vi "Test-FAMM.vi"() -> ()   [LabVIEW 2014, in "FAMM.lvclass"]
doc: "Test the Historian performance"
uses:
  FAMM.lvclass
  HISW/HISW.lvclass
  FAMM.lvclass/FAMM.ctl
  Common/controls/GlobalClassRefs.vi
panel:
  out "Tags":i32
  out "error out":errorcluster
  out "Database Class":string
  out "FAMM_PAQ_Layers":i32
  out "37x37":picture
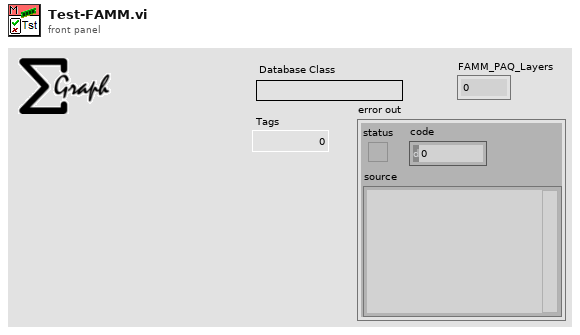
[diagram p1: front panel]
types:
  T1 = typedef "typedef_PAQsample.ctl" = cluster{"TAGs":string[], "status":u32[], "data":dbl[], "Source":string[]}
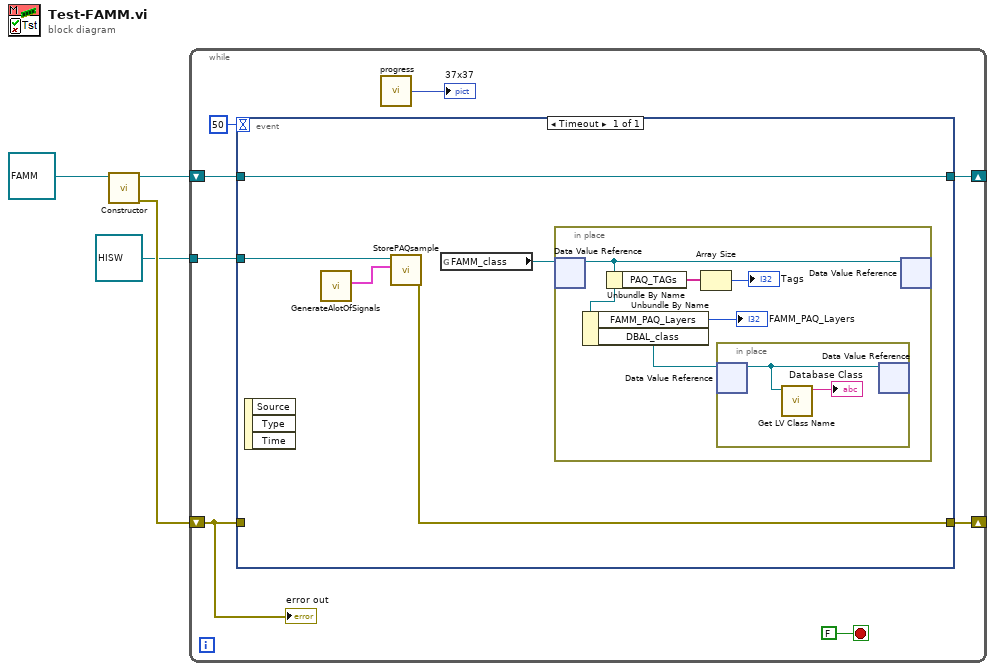
[diagram p0: block diagram]
diagram:
  n1 = call "Constructor.vi"("FAMM in"=refnum<class "FAMM.lvclass"> refnum) -> ("error out"=w4:errorcluster, "FAMM out"=w1:refnum<class "FAMM.lvclass">)  [unwired: 9 in]
  n2 = while {
    shift-right: [w9] -> _
    shift-left: w1 -> [w10]
    shift-right: [w8] -> _
    shift-left: w4 -> [w5]
    tunnel: refnum<class "HISW.lvclass"> refnum ("HISW in") -> [w6]
    stop <- FALSE stop-if-true
    n3 = event shown="[0] Timeout" {
      selector: _ -> [_]
      dyn-events: _ -> [_]
      timeout: 50 -> [_]
      tunnel: w10 -> [w14]
      tunnel: [w14] -> w9
      tunnel: w5 -> [_]
      tunnel: [w16] -> w8
      tunnel: w6 -> [w15]
      event Timeout {
        n4 = event-data() -> ()  [unwired: 1 in, 3 out]
        n5 = call "GenerateAlotOfSignals.vi"() -> ("DAQ"=w17:T1)  [unwired: 11 in]
        n6 = call "StorePAQsample.vi"("PAQ IN"=w17, "HISW in"=w15) -> ("error out"=w16:errorcluster)  [unwired: 8 in, 1 out]
        n7 = global read "GlobalClassRefs.vi" "FAMM_class"() -> (w13:refnum<data-value>)
        n8 = in-place {
          n9 = in-place-dvr #1(w13) -> (w19:refnum<class "FAMM.lvclass">)  [unwired: 1 out]
          n10 = Unbundle By Name(w19) -> ("FAMM_PAQ_Layers"=→"FAMM_PAQ_Layers":i32, "DBAL_class"=w18:refnum<data-value>)
          n11 = Unbundle By Name(w19) -> ("PAQ_TAGs"=w22:string[])
          n12 = Array Size(array=w22) -> (size(s)=→"Tags":i32)
          n13 = in-place {
            n14 = in-place-dvr #2(w18) -> (w24:refnum<class "DBAL.lvclass">)  [unwired: 1 out]
            n15 = call <vilib>:"Get LV Class Name.vi"("object"=w24) -> ("class name"=→"Database Class":string)  [unwired: 9 in, 1 out]
            n16 = in-place-dvr #2(w24) -> ()  [unwired: 2 out]
          }
          n17 = in-place-dvr #1(w19) -> ()  [unwired: 2 out]
        }
      }
    }
    n18 = call "progress.vi"() -> ("37x37"=→"37x37":picture)  [unwired: 7 in]
    "error out" <- w5
  }
